vi "Launch Pane Relief.vi"(8 "error in (no error)":errorcluster, 9 "Undo Transaction Name":string="PaneRelief", 11 "VI in":refnum<vi>) -> (0 "error out":errorcluster, 3 "VI out":refnum<vi>)   [LabVIEW 2015]
uses:
  Typedefs/Selection Colors--Cluster.ctl
  <vilib>/MGI/Panel Manager/Panel/Window Position/Persistent Position/Persistent Position.vi
  <vilib>/MGI/Panel Manager/Panel Actor/Panel Actor/Launch Root Panel Window.vi
  Classes/Pane Relief Main UI/Pane Relief Main UI/Pane Relief Main UI.lvclass
  <vilib>/MGI/Panel Manager/Panel Actor/Panel Actor/Panel Actor.lvclass
  <vilib>/MGI/Panel Manager/Panel/Panel.lvlib
  <vilib>/MGI/Panel Manager/Panel/Window Position/Persistent Position/Persistent Position.lvclass
  <vilib>/MGI/Monitored Actor/Monitored Actor.lvlib
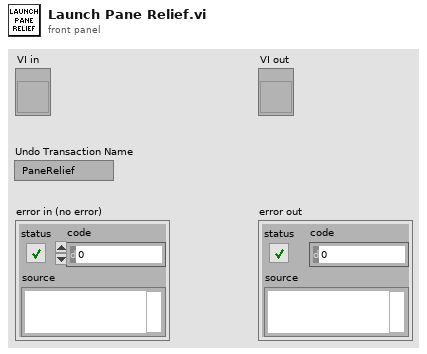
[diagram p1: front panel]
types:
  T1 = typedef "Selection Colors--Cluster.ctl" = cluster{"Normal":u32, "Mouse-over":u32, "Selected":u32, "Selected Mouse-over":u32}
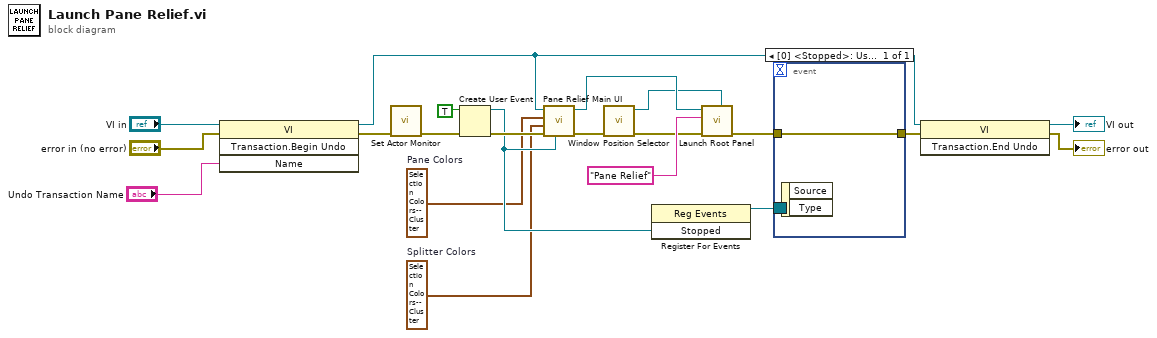
[diagram p0: block diagram]
diagram:
  w3 = T1 {"Normal"=13620442, "Mouse-over"=12304582, "Selected"=3245000, "Selected Mouse-over"=1011636}  # Pane Colors
  w2 = T1 {"Normal"=8818326, "Mouse-over"=7502466, "Selected"=1994152, "Selected Mouse-over"=741250}  # Splitter Colors
  n1 = invoke class="VI" method="Transaction.Begin Undo"(reference="VI in", error in="error in (no error)", "Name"="Undo Transaction Name") -> (reference out=w1:refnum<vi>, error out=w6:errorcluster)  [unwired: 1 in, 2 out]
  n2 = call <vilib>:"Set Actor Monitor.vi"("error in (no error)"=w6) -> ("error out"=w5:errorcluster)  [unwired: 10 in]
  n3 = Create User Event(user event datatype=TRUE ("Stopped"), error in=w5) -> (user event=w4:refnum<user-event>, error out=w10:errorcluster)
  n4 = call "Pane Relief Main UI.vi"("Stopped Event"=w4, "Error In"=w10, "Splitter Colors"=w2, "Pane Colors"=w3, "QD Launch VI Ref"=w1) -> ("Error Out"=w13:errorcluster, "Pane Relief Main UI out"=w16:refnum<class "Pane Relief Main UI.lvclass">)  [unwired: 5 in]
  n5 = call-poly <vilib>:"Window Position Selector.vi"("Error In"=w13) -> ("Error Out"=w12:errorcluster, "Persistent Position out"=w15:refnum<class "Window Position.lvclass">)  [unwired: 9 in]
  n6 = register-events(w4) -> (reference out=w7:refnum<event-registration>)  [unwired: 2 in, 1 out]
  n7 = call-poly <vilib>:"Launch Root Panel.vi"("Window Position (Maximize First Call)"=w15, "Error In"=w12, "Title"="Pane Relief", "Panel Actor in"=w16) -> ("Error Out"=w8:errorcluster)  [unwired: 6 in, 1 out]
  n8 = event shown="[0] <Stopped>: User Event" {
    selector: w7 -> [_]
    dyn-events: _ -> [_]
    timeout: _ -> [_]
    tunnel: [w22] -> w9
    tunnel: w8 -> [w22]
    event User Event {
      n9 = event-data() -> ()  [unwired: 1 in, 2 out]
    }
  }
  n10 = invoke class="VI" method="Transaction.End Undo"(reference=w1, error in=w9) -> (reference out=→"VI out":refnum<vi>, error out=→"error out":errorcluster)  [unwired: 1 in, 1 out]
